vi "RGB Color.vi"(8 "error in (no error)":errorcluster, 10 "Color":u32(colorbox), 11 "Color in":refnum<class "Color.lvclass">) -> (0 "error out":errorcluster, 3 "Color out":refnum<class "Color.lvclass">)   [LabVIEW 2016, in "DataGrid.lvlib" / "Color.lvclass"]
doc: "Sets the color class according to a colorbox input, for determining the RGB color values of the class. Use Set Alpha property separately if you want transparency."
uses:
  <userlib>/LabVIEWdotNetDataGrid/source/Color/Color.lvclass
  System.Drawing
  <userlib>/LabVIEWdotNetDataGrid/source/Color/Color.lvclass/Color.ctl
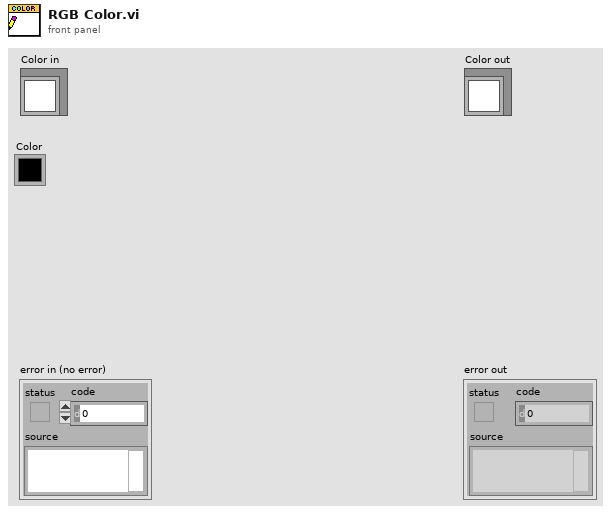
[diagram p1: front panel]
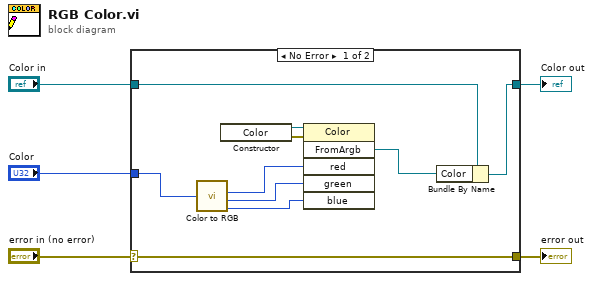
[diagram p0: block diagram]
diagram:
  n1 = case shown="No Error" "error in (no error)" {
    selector: "error in (no error)" -> [w15 w16]
    tunnel: [w15 w16] -> w4
    tunnel: [w14 w17] -> w2
    tunnel: "Color in" -> [w6 w17]
    tunnel: "Color" -> [w11 _]
    frame No Error {
      n2 = call <vilib>:"Color to RGB.vi"("Color"=w11) -> ("R"=w10:u8, "G"=w9:u8, "B"=w8:u8)  [unwired: 1 out]
      n3 = constructor class="Color"() -> (reference out=w13:refnum<k24>, error out=w12:errorcluster)  [unwired: 3 in, 1 out]
      n4 = invoke class="Color" method="FromArgb"(reference=w13, error in=w12, "red"=w10, "green"=w9, "blue"=w8) -> ("FromArgb"=w7:refnum<k24>)  [unwired: 1 in, 5 out]
      n5 = Bundle By Name(cluster=w6, "Color"=w7) -> (w14:refnum<class "Color.lvclass">)
    }
    frame Error {
    }
  }
  "error out" <- w4
  "Color out" <- w2
